vi "DataProcess_JointTorque.vi"() -> ()   [LabVIEW 2016]
uses:
  <vilib>/Utility/file.llb/Write Delimited Spreadsheet (DBL).vi
  <vilib>/AuZn/auzn custom VIs/AuZnCustomVI.lvlib
panel:
  in  "Output Path":path
  out "File Name":string
  out "Total":i32
  out "Current":i32
  in  "pattern":string
  in  "Path":path
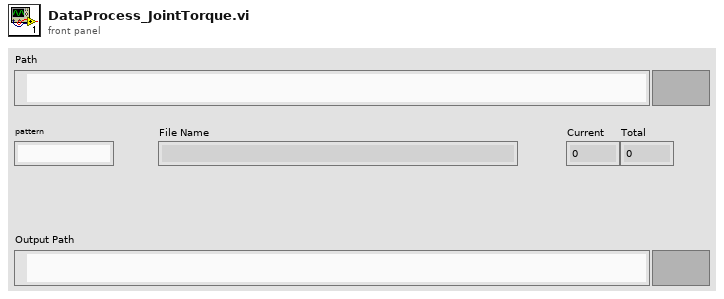
[diagram p1: front panel]
types:
  T1 = enum16{"open", "replace", "create", "open or create", "replace or create", "replace or create with confirmation"}
  T2 = cluster{"Desired_Mean":dbl[][], "Desired_Std":dbl[][], "Plan_Mean":dbl[][], "Plan_Std":dbl[][], "Actual_Mean":dbl[][], "Actual_Std":dbl[][]}
  T3 = cluster{"All Error":dbl[], "Planning Error":dbl[], "PID Error":dbl[]}
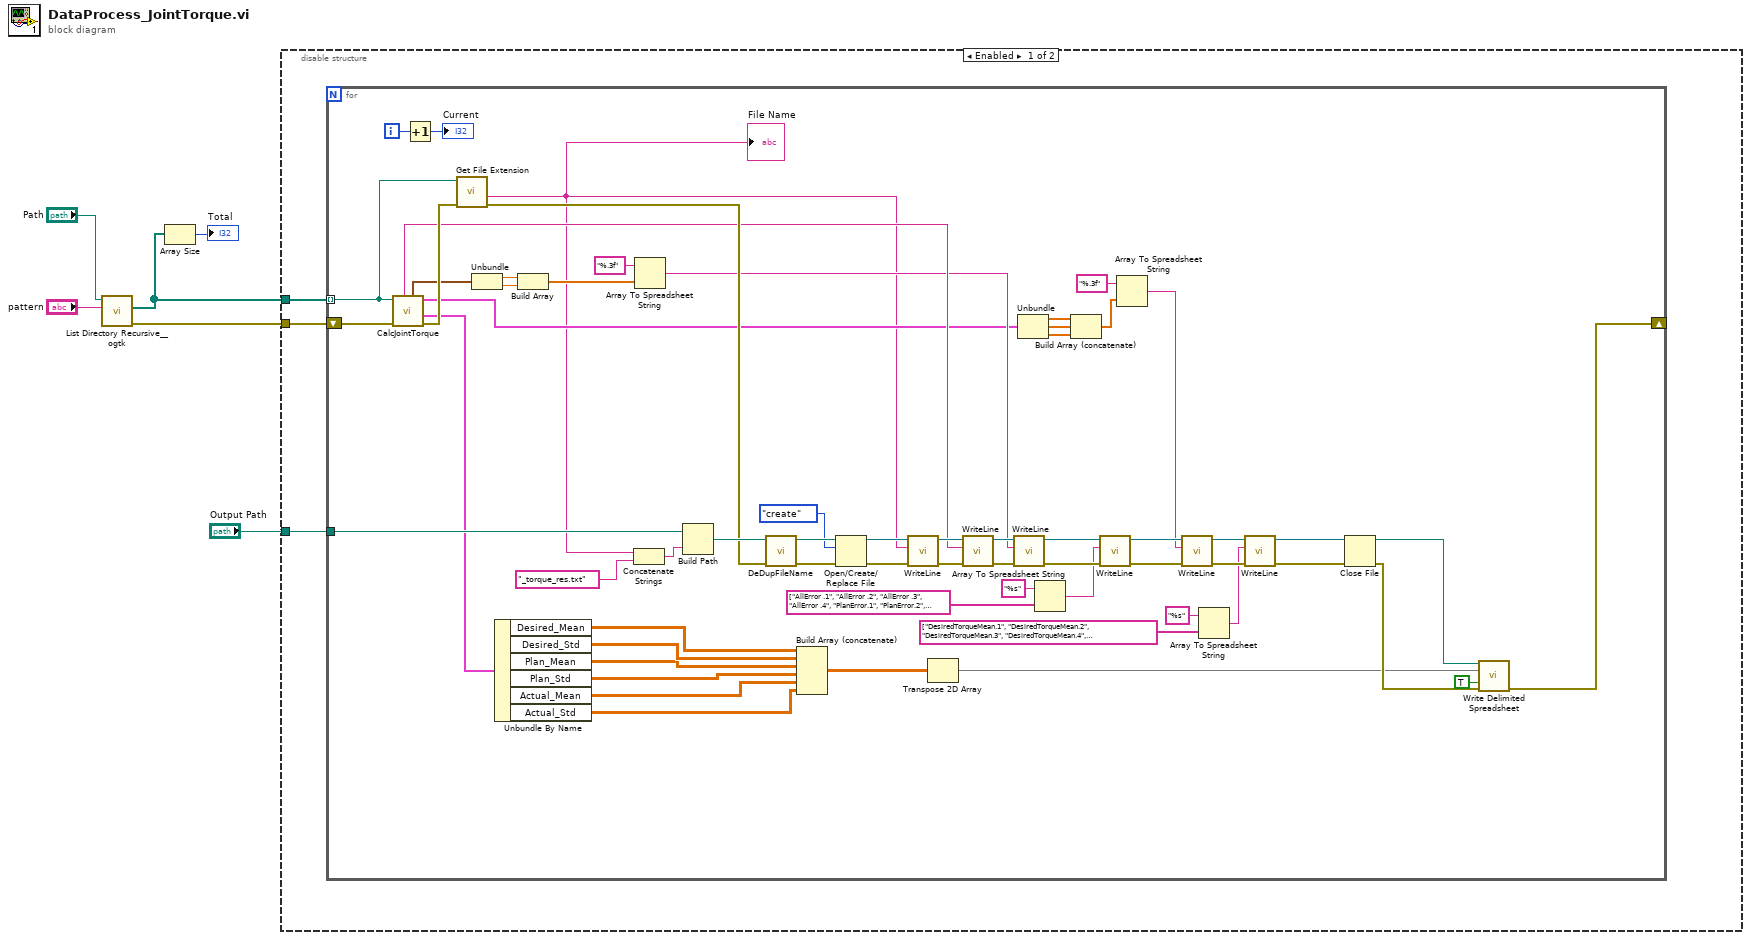
[diagram p0: block diagram]
diagram:
  n1 = call <userlib>:"List Directory Recursive__ogtk.vi"("pattern"="pattern", "Path"="Path") -> ("error out"=w1:errorcluster, "file paths"=w4:path[])  [unwired: 6 in, 2 out]
  n2 = Array Size(array=w4) -> (size(s)=→"Total":i32)
  n3 = disable-structure shown="Enabled" {
    disable-tunnel: w4 -> [w9 _]
    disable-tunnel: "Output Path" -> [w8 _]
    disable-tunnel: w1 -> [w7 _]
    frame Enabled {
      n4 = for {
        tunnel: w9 -> [w67] mode=indexing
        tunnel: w8 -> [w47]
        shift-right: [w38] -> _
        shift-left: w7 -> [w37]
        i -> [w70]
        n5 = call "CalcJointTorque.vi"("error in (no error)"=w37, "Path"=w67) -> ("error out"=w66:errorcluster, "AverageTorque"=w17:T2, "Torque Errors"=w36:T3, "ExtraWeight(kg)"=w51:cluster{"Thigh":dbl, "Shank":dbl}, "match substring"=w54:string)  [unwired: 4 in, 1 out]
        n6 = Increment(x=w70) -> (x+1=→"Current":i32)
        n7 = call <vilib>:"Get File Extension.vi"("error in (no error)"=w66, "file"=w67) -> ("error out"=w62:errorcluster, "filename without extension"=w18:string)  [unwired: 5 in, 3 out]
        "File Name" <- w18
        n8 = Unbundle(w51) -> ("Thigh"=w49:dbl, "Shank"=w50:dbl)
        n9 = Unbundle By Name(w17) -> ("Desired_Mean"=w16:dbl[][], "Desired_Std"=w15:dbl[][], "Plan_Mean"=w14:dbl[][], "Plan_Std"=w13:dbl[][], "Actual_Mean"=w12:dbl[][], "Actual_Std"=w11:dbl[][])
        n10 = Build Array(w49, w50) -> (w48:dbl[])
        n11 = Concatenate Strings(w18, "_torque_res.txt" ("string")) -> (w65:string)
        n12 = Array To Spreadsheet String(array=w48, 3:"%.3f" ("format string")) -> (spreadsheet string=w46:string)  [unwired: 1 in]
        n13 = Build Path(base path=w47, name or relative path=w65) -> (appended path=w63:path)
        n14 = call <vilib>:"DeDupFileName.vi"("error in (no error)"=w62, "Path"=w63) -> ("error out"=w61:errorcluster, "Out Path"=w60:path)  [unwired: 7 in, 1 out]
        n15 = Build Array (concatenate)(w16, w15, w14, w13, w12, w11) -> (w68:dbl[][])
        n16 = Open/Create/Replace File(file path (use dialog)=w60, error in=w61, operation (0:open)=T1."create") -> (refnum out=w58:refnum<file>, error out=w55:errorcluster)  [unwired: 3 in, 1 out]
        n17 = call <vilib>:"WriteLine.vi"("error in (no error)"=w55, "text"=w18, "refnum in"=w58) -> ("error out"=w57:errorcluster, "refnum out"=w56:refnum<file>)  [unwired: 6 in, 1 out]
        n18 = Transpose 2D Array(2D array=w68) -> (transposed array=w19:dbl[][])
        n19 = call <vilib>:"WriteLine.vi"("error in (no error)"=w57, "text"=w54, "refnum in"=w56) -> ("error out"=w53:errorcluster, "refnum out"=w52:refnum<file>)  [unwired: 6 in, 1 out]
        n20 = call <vilib>:"WriteLine.vi"("error in (no error)"=w53, "text"=w46, "refnum in"=w52) -> ("error out"=w44:errorcluster, "refnum out"=w43:refnum<file>)  [unwired: 6 in, 1 out]
        n21 = Unbundle(w36) -> ("All Error"=w28:dbl[], "Planning Error"=w27:dbl[], "PID Error"=w26:dbl[])
        n22 = Array To Spreadsheet String(array=string[] ["AllError .1", "AllError .2", "AllError .3", "AllError .4", "PlanError.1", "PlanError.2", "PlanError.3", "PlanError.4", "PIDError.1", "PIDError.2", "PIDError.3", "PIDError.4"] ("Array"), 3:"%s" ("format string")) -> (spreadsheet string=w21:string)  [unwired: 1 in]
        n23 = Build Array (concatenate)(w28, w27, w26) -> (w24:dbl[])
        n24 = call <vilib>:"WriteLine.vi"("error in (no error)"=w44, "text"=w21, "refnum in"=w43) -> ("error out"=w35:errorcluster, "refnum out"=w32:refnum<file>)  [unwired: 6 in, 1 out]
        n25 = Array To Spreadsheet String(array=w24, 3:"%.3f" ("format string")) -> (spreadsheet string=w23:string)  [unwired: 1 in]
        n26 = call <vilib>:"WriteLine.vi"("error in (no error)"=w35, "text"=w23, "refnum in"=w32) -> ("error out"=w34:errorcluster, "refnum out"=w31:refnum<file>)  [unwired: 6 in, 1 out]
        n27 = Array To Spreadsheet String(array=string[] ["DesiredTorqueMean.1", "DesiredTorqueMean.2", "DesiredTorqueMean.3", "DesiredTorqueMean.4", "DesiredTorqueStd.1", "DesiredTorqueStd.2", "DesiredTorqueStd.3", "DesiredTorqueStd.4", "PlannedTorqueMean.1", "PlannedTorqueMean.2", "PlannedTorqueMean.3", "PlannedTorqueMean.4", "PlannedTorqueStd.1", "PlannedTorqueStd.2", "PlannedTorqueStd.3", "PlannedTorqueStd.4", "ActuralTorqueMean.1", "ActuralTorqueMean.2", "ActuralTorqueMean.3", "ActuralTorqueMean.4", "ActuralTorqueStd.1", "ActuralTorqueStd.2", "ActuralTorqueStd.3", "ActuralTorqueStd.4", ""], 3:"%s" ("format string")) -> (spreadsheet string=w29:string)  [unwired: 1 in]
        n28 = call <vilib>:"WriteLine.vi"("error in (no error)"=w34, "text"=w29, "refnum in"=w31) -> ("error out"=w33:errorcluster, "refnum out"=w30:refnum<file>)  [unwired: 6 in, 1 out]
        n29 = Close File(refnum=w30, error in=w33) -> (path=w41:path, error out=w40:errorcluster)
        n30 = call-poly <vilib>:"Write Delimited Spreadsheet.vi"("file path (dialog if empty)"=w41, "2D data"=w19, "append to file? (new file:F)"=TRUE ("append to file? (F)"), "error in (no error)"=w40) -> ("error out"=w38:errorcluster)  [unwired: 10 in, 1 out]
      }
    }
    frame Disabled {
    }
  }
